vi "Set PCL Timing Source.vi"(8 "error in (no error)":errorcluster, 10 "Timing Source":enum16{"Automatic", "Custom Device"}(ring), 11 "Item Ref in":T1 format="%.0x") -> (0 "error out":errorcluster, 3 "Item Ref out":T1 format="%.0x")   [LabVIEW 2010, in "PXIe-433x Custom Device.lvlib"]
uses:
  PXIe-433x Custom Device.lvlib
  <vilib>/NI Veristand/Custom Device API/Custom Device Item Ref.ctl
  NationalInstruments.VeriStand.SystemStorage
  <vilib>/NI Veristand/Custom Device Tools/Custom Device Utility Library/Custom Device Utility Library.lvlib
  <vilib>/NI Veristand/Custom Device API/Custom Device API.lvlib
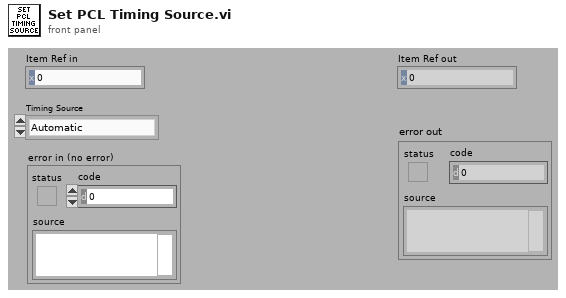
[diagram p1: front panel]
types:
  T1 = typedef "Custom Device API.lvlib/Custom Device Item Ref.ctl" = u64
  T2 = typedef "Custom Device API.lvlib/Custom Device Pointer.ctl" = refnum<k24>
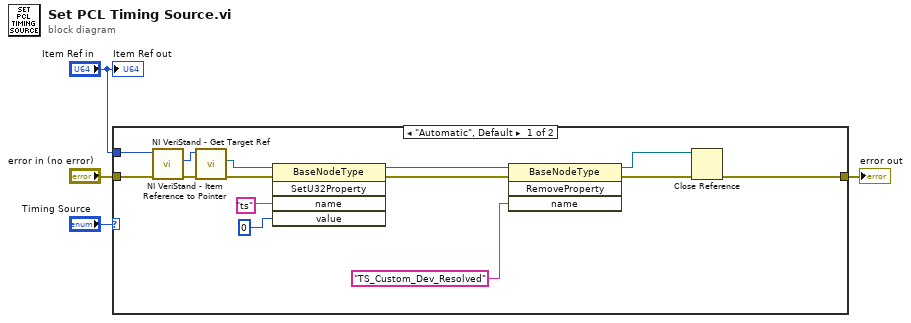
[diagram p0: block diagram]
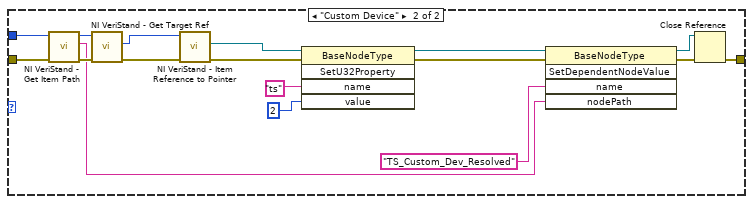
[diagram p2: hidden frame]
diagram:
  n1 = case shown="\"Automatic\", Default" "Timing Source" {
    tunnel: "Item Ref in" -> [w17 w35]
    tunnel: "error in (no error)" -> [w18 w34]
    tunnel: [w5 w19] -> w2
    frame "Automatic", Default {
      n2 = call <vilib>:"NI VeriStand - Get Target Ref.vi"("error in"=w18, "Item Ref in"=w17) -> ("error out"=w16:errorcluster, "Target Ref"=w15:T1)  [unwired: 6 in, 2 out]
      n3 = call <vilib>:"NI VeriStand - Item Reference to Pointer.vi"("error in (no error)"=w16, "Item Ref in"=w15) -> ("error out"=w14:errorcluster, "Node Pointer"=w13:T2)  [unwired: 6 in, 2 out]
      n4 = invoke class="BaseNodeType" method="SetU32Property"(reference=w13, error in=w14, "name"="ts", "value"=u32 0) -> (reference out=w9:T2, error out=w10:errorcluster)  [unwired: 1 in, 3 out]
      n5 = invoke class="BaseNodeType" method="RemoveProperty"(reference=w9, error in=w10, "name"="TS_Custom_Dev_Resolved") -> (reference out=w7:T2, error out=w6:errorcluster)  [unwired: 1 in, 2 out]
      n6 = Close Reference(reference=w7, error in (no error)=w6) -> (error out=w5:errorcluster)
    }
    frame "Custom Device" {
      n7 = call <vilib>:"NI VeriStand - Get Item Path.vi"("error in (no error)"=w34, "Item Ref in"=w35) -> ("error out"=w33:errorcluster, "Path"=w23:string, "Item Ref out"=w32:T1)  [unwired: 6 in, 1 out]
      n8 = call <vilib>:"NI VeriStand - Get Target Ref.vi"("error in"=w33, "Item Ref in"=w32) -> ("error out"=w31:errorcluster, "Target Ref"=w30:T1)  [unwired: 6 in, 2 out]
      n9 = call <vilib>:"NI VeriStand - Item Reference to Pointer.vi"("error in (no error)"=w31, "Item Ref in"=w30) -> ("error out"=w26:errorcluster, "Node Pointer"=w29:T2)  [unwired: 6 in, 2 out]
      n10 = invoke class="BaseNodeType" method="SetU32Property"(reference=w29, error in=w26, "name"="ts", "value"=u32 2) -> (reference out=w24:T2, error out=w25:errorcluster)  [unwired: 1 in, 3 out]
      n11 = invoke class="BaseNodeType" method="SetDependentNodeValue"(reference=w24, error in=w25, "name"="TS_Custom_Dev_Resolved", "nodePath"=w23) -> (reference out=w21:T2, error out=w20:errorcluster)  [unwired: 1 in, 3 out]
      n12 = Close Reference(reference=w21, error in (no error)=w20) -> (error out=w19:errorcluster)
    }
  }
  "error out" <- w2
  "Item Ref out" <- "Item Ref in"
